vi "Interpolate Parameter.vi"(8 "error in (no error)":errorcluster, 10 "Parameter-array":dbl[](array[numeric]) format="%.2p", 11 "XY-data":cluster{"X-array":dbl[], "Y-array":dbl[]}[](array[cluster]) {"Y-array" format="%.2p"; "X-array" format="%.2p"}) -> (0 "error out":errorcluster, 2 "Interpolated Parameter-array":dbl[](array[numeric]), 3 "Interpolated XY-data out":cluster{"X-array":dbl[], "Y-array":dbl[]}[](array[cluster]) {"Y-array" format="%.2p"; "X-array" format="%.2p"})   [LabVIEW 2016, in "xy_utilities.lvlib"]
doc: "Interpolate the input <b>XY-data</b> along the <b>Parameter-array</b> axis."
uses:
  xy_utilities.lvlib
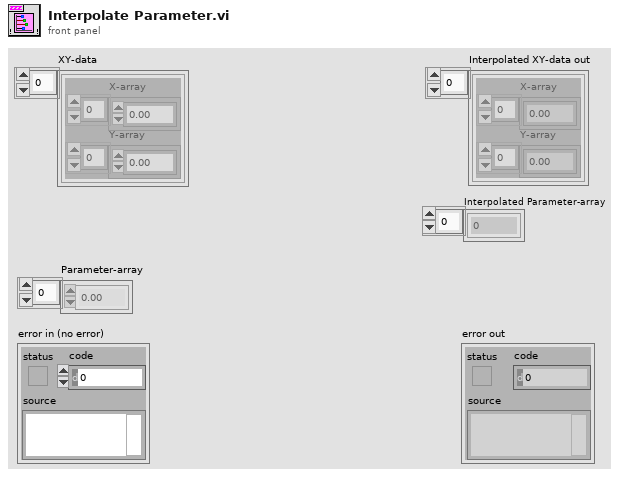
[diagram p1: front panel]
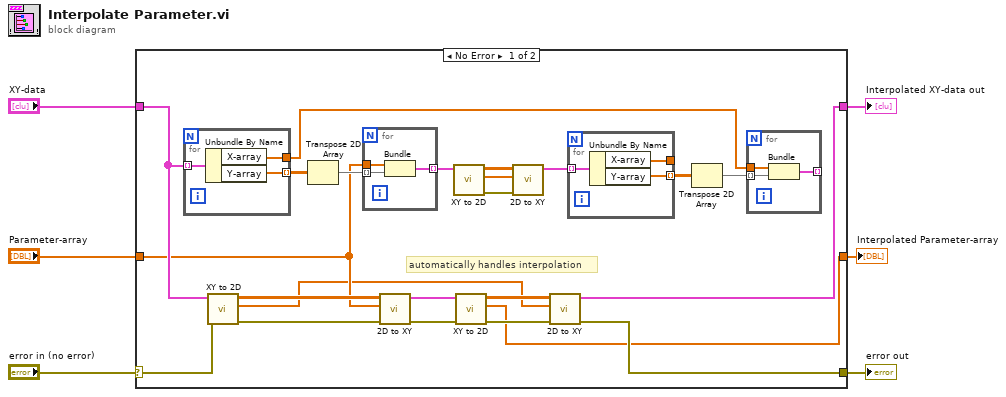
[diagram p0: block diagram]
diagram:
  n1 = case shown="No Error" "error in (no error)" {
    selector: "error in (no error)" -> [w13 w44]
    tunnel: "XY-data" -> [w19 w43]
    tunnel: [w8 w43] -> w4
    tunnel: [w9 w44] -> w3
    tunnel: "Parameter-array" -> [w17 w42]
    tunnel: [w7 w42] -> w1
    frame No Error {
      # "automatically handles interpolation"
      n2 = for {
        tunnel: w19 -> [w41] mode=indexing
        tunnel: [w40] -> w29 mode=indexing
        tunnel: [w39] -> w25
        n3 = Unbundle By Name(w41) -> ("X-array"=w39:dbl[], "Y-array"=w40:dbl[])
      }
      n4 = call "XY to 2D.vi"("error in (no error)"=w13, "XY-data"=w19) -> ("error out"=w12:errorcluster, "X Array"=w14:dbl[], "2D Y Array"=w18:dbl[][])  [unwired: 7 in]
      n5 = Transpose 2D Array(2D array=w29) -> (transposed array=w28:dbl[][])
      n6 = for {
        tunnel: w28 -> [w38] mode=indexing
        tunnel: w17 -> [w37]
        tunnel: [w36] -> w21 mode=indexing
        n7 = Bundle("Parameter-array"=w37, w38) -> (w36:cluster{"Parameter-array":dbl[], dbl[]})  [unwired: 1 in]
      }
      n8 = call "2D to XY.vi"("error in (no error)"=w12, "X Array"=w17, "2D Y Array"=w18) -> ("error out"=w11:errorcluster, "XY-data out"=w16:cluster{"X-array":dbl[], "Y-array":dbl[]}[])  [unwired: 7 in]
      n9 = call "XY to 2D.vi"("XY-data"=w21) -> ("error out"=w22:errorcluster, "X Array"=w23:dbl[], "2D Y Array"=w24:dbl[][])  [unwired: 8 in]
      n10 = call "XY to 2D.vi"("error in (no error)"=w11, "XY-data"=w16) -> ("error out"=w10:errorcluster, "X Array"=w7:dbl[], "2D Y Array"=w15:dbl[][])  [unwired: 7 in]
      n11 = call "2D to XY.vi"("error in (no error)"=w22, "X Array"=w23, "2D Y Array"=w24) -> ("XY-data out"=w20:cluster{"X-array":dbl[], "Y-array":dbl[]}[])  [unwired: 7 in, 1 out]
      n12 = call "2D to XY.vi"("error in (no error)"=w10, "X Array"=w14, "2D Y Array"=w15) -> ("error out"=w9:errorcluster, "XY-data out"=w8:cluster{"X-array":dbl[], "Y-array":dbl[]}[])  [unwired: 7 in]
      n13 = for {
        tunnel: w20 -> [w35] mode=indexing
        tunnel: [w34] -> w26 mode=indexing
        tunnel: [w33] -> _
        n14 = Unbundle By Name(w35) -> ("X-array"=w33:dbl[], "Y-array"=w34:dbl[])
      }
      n15 = Transpose 2D Array(2D array=w26) -> (transposed array=w27:dbl[][])
      n16 = for {
        tunnel: w27 -> [w32] mode=indexing
        tunnel: w25 -> [w31]
        tunnel: [w30] -> _ mode=indexing
        n17 = Bundle("X-array"=w31, w32) -> (w30:cluster{"X-array":dbl[], dbl[]})  [unwired: 1 in]
      }
    }
    frame Error {
    }
  }
  "error out" <- w3
  "Interpolated XY-data out" <- w4
  "Interpolated Parameter-array" <- w1
